vi "Is part of a project.vi"(8 "error in (no error)":errorcluster, 11 "VI Reference":refnum<vi>) -> (0 "error out":errorcluster, 3 "Is part of a project":bool)   [LabVIEW 2021]
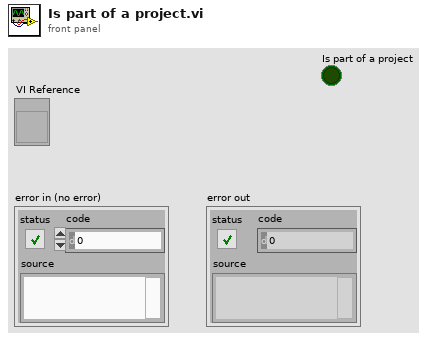
[diagram p1: front panel]
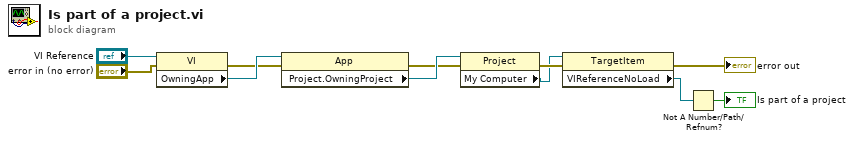
[diagram p0: block diagram]
diagram:
  n1 = property class="VI"(reference="VI Reference", error in="error in (no error)") -> (error out=w8:errorcluster, "OwningApp"=w10:refnum<vi>)  [unwired: 1 out]
  n2 = property class="App"(reference=w10, error in=w8) -> (error out=w7:errorcluster, "Project.OwningProject"=w9:refnum<vi>)  [unwired: 1 out]
  n3 = property class="Project"(reference=w9, error in=w7) -> (error out=w4:errorcluster, "My Computer"=w3:refnum<vi>)  [unwired: 1 out]
  n4 = property class="TargetItem"(reference=w3, error in=w4) -> (error out=→"error out":errorcluster, "VIReferenceNoLoad"=w2:refnum<vi>)  [unwired: 1 out]
  n5 = Not A Number/Path/Refnum?(number/path/refnum=w2) -> (NaN/Path/Refnum?=→"Is part of a project":bool)
